vi "Populate Single Control.vi"(5 "Clust Refnum":refnum<vi>, 6 "VI Refnum":refnum<vi>, 7 "Prefix":string, 8 "error in (no error)":errorcluster, 9 "Values":string[](array[string]), 10 "Keys":string[](array[string]), 11 "Ctl Refnum":refnum<vi>) -> (0 "error out":errorcluster, 1 "Variant":variant, 3 "Ctl Refnum out":refnum<vi>, 4 "VI Refnum out":refnum<vi>)   [LabVIEW 2018]
panel:
  in  "type specifier":refnum<vi>
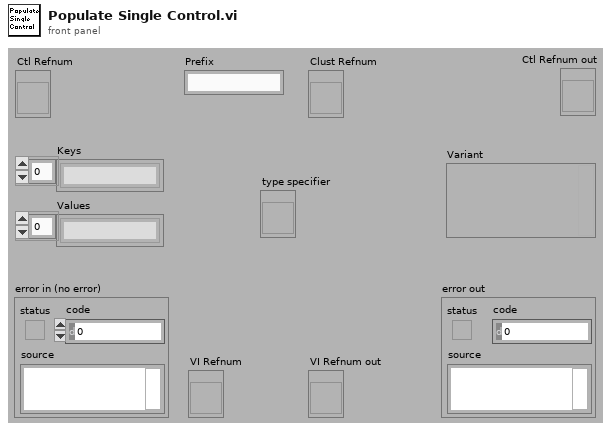
[diagram p1: front panel]
types:
  T1 = typedef "LVComboBoxStrsAndValuesArrayTypeDef.ctl" = cluster{"String":string, "Value":string}[]
  T2 = typedef "LVStringsAndValuesArrayTypeDef.ctl" = cluster{"String":string, "Value":ext}[]
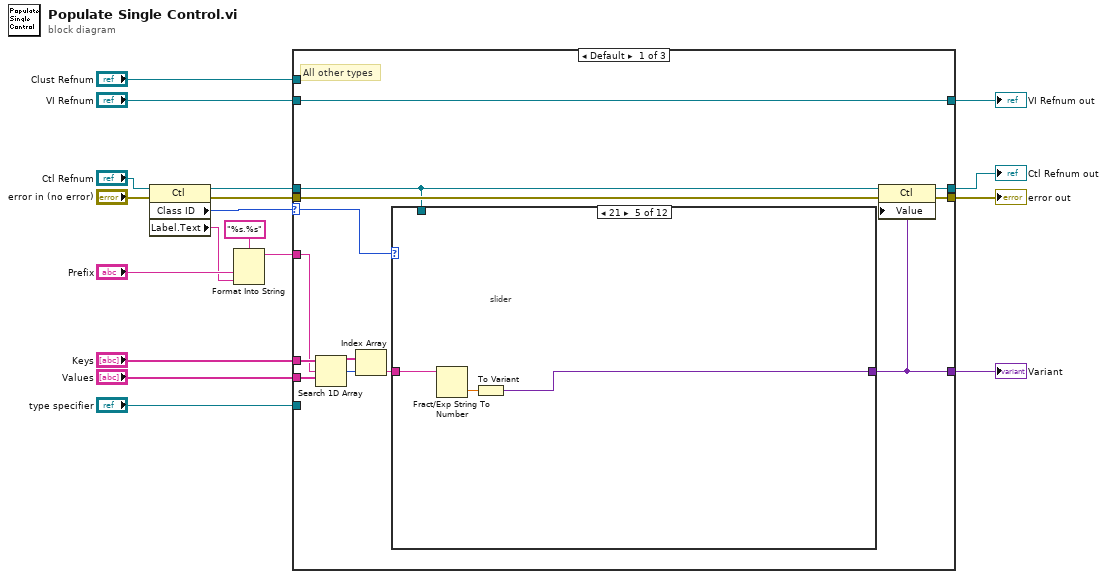
[diagram p0: block diagram]
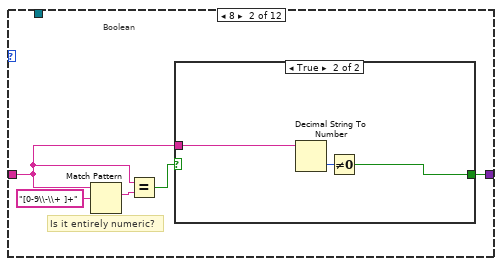
[diagram p3: hidden frame]
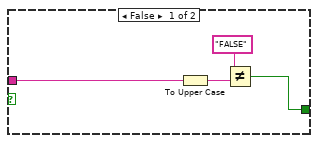
[diagram p4: hidden frame]
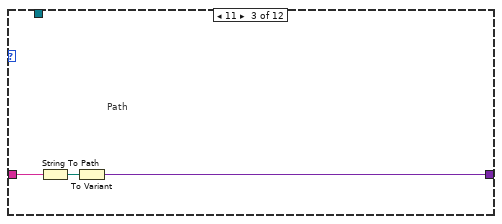
[diagram p5: hidden frame]
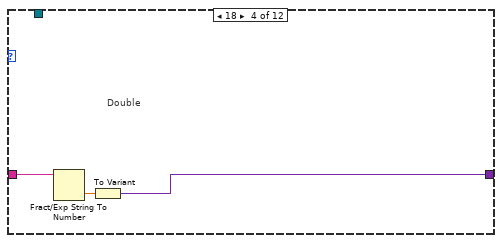
[diagram p6: hidden frame]
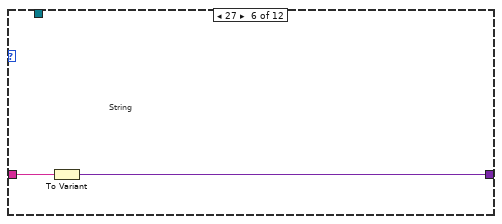
[diagram p7: hidden frame]
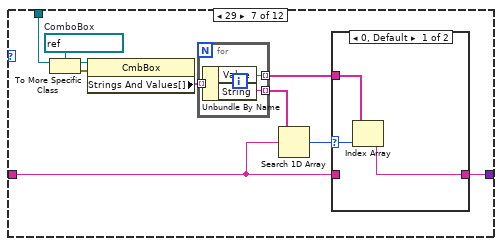
[diagram p8: hidden frame]
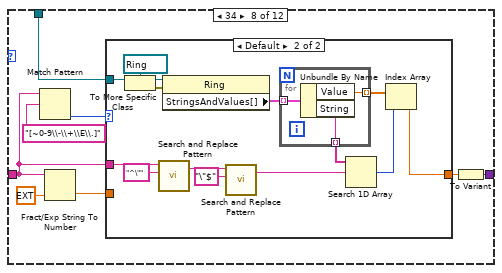
[diagram p10: hidden frame]
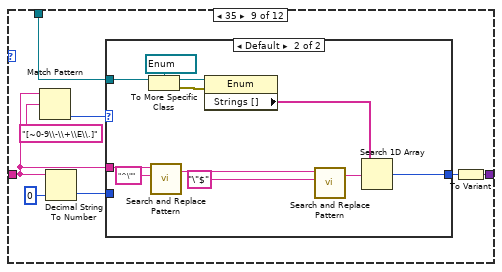
[diagram p12: hidden frame]
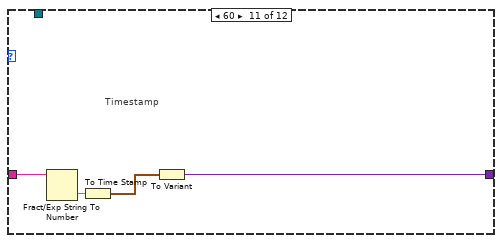
[diagram p15: hidden frame]
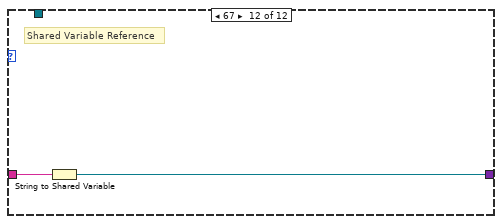
[diagram p16: hidden frame]
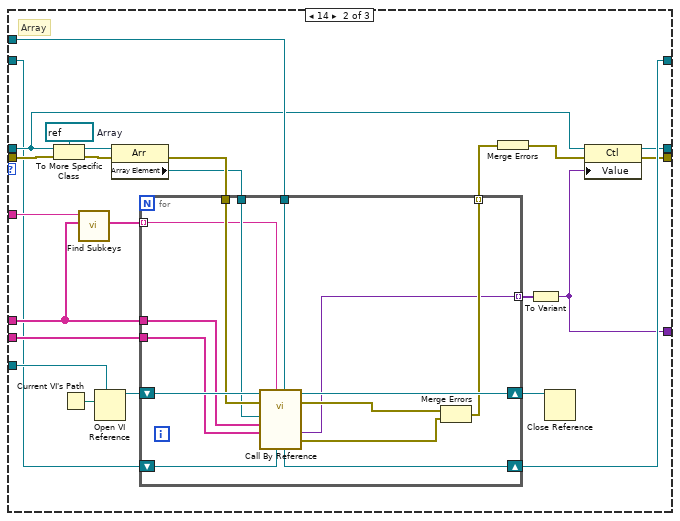
[diagram p17: hidden frame]
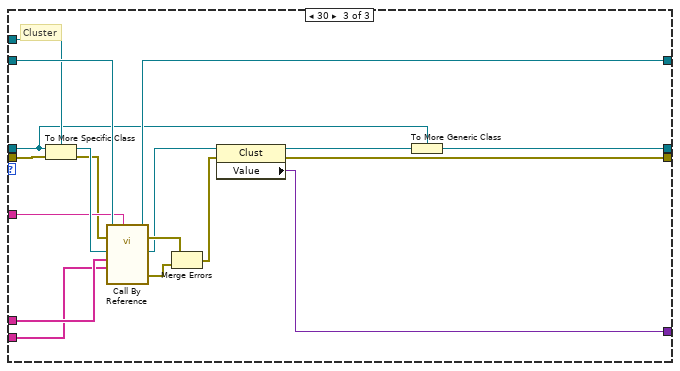
[diagram p18: hidden frame]
diagram:
  n1 = property class="Ctl"(reference="Ctl Refnum", error in="error in (no error)") -> (reference out=w10:refnum<vi>, error out=w11:errorcluster, "Class ID"=w9:u32, "Label.Text"=w6:string)
  n2 = Format Into String(format string="%s.%s", "Prefix", w6) -> (resulting string=w18:string)  [unwired: 2 in, 1 out]
  n3 = case shown="Default" w9 {
    selector: w9 -> [w25 _ _]
    tunnel: "VI Refnum" -> [w26 w125 w178]
    tunnel: w10 -> [w20 w135 w170]
    tunnel: w11 -> [w29 w147 w179]
    tunnel: w18 -> [w19 w132 w173]
    tunnel: "Values" -> [w30 w143 w175]
    tunnel: "Keys" -> [w23 w131 w176]
    tunnel: [w26 w144 w177] -> w14
    tunnel: [w28 w134 w171] -> w17
    tunnel: [w27 w126 w162] -> w16
    tunnel: "Clust Refnum" -> [_ w145 w172]
    tunnel: [w21 w133 w165] -> w3
    tunnel: "type specifier" -> [_ w138 _]
    frame Default {
      # "All other types"
      n4 = Search 1D Array(1D array=w23, element=w19) -> (index of element=w22:i32)  [unwired: 1 in]
      n5 = Index Array(array=w30, index=w22) -> (element=w24:string)
      n6 = case shown="21" w25 {
        tunnel: w24 -> [_ w31 w44 w48 w51 w52 w56 w71 w97 w117 w121 w123]
        tunnel: [_ w32 w45 w46 w49 w53 w55 w77 w103 w117 w120 w122] -> w21
        tunnel: w20 -> [_ _ _ _ _ _ w63 w76 w102 _ _ _]
        frame Default {
        }
        frame 8 {
          # "Is it entirely numeric?"
          # "Boolean"
          n7 = Match Pattern(string=w31, regular expression="[0-9\\-\\+ ]+") -> (match substring=w34:string)  [unwired: 1 in, 3 out]
          n8 = Equal?(x=w31, y=w34) -> (x = y?=w33:bool)
          n9 = case shown="True" w33 {
            tunnel: [w36 w40] -> w32
            tunnel: w31 -> [w37 w42]
            frame False {
              n10 = To Upper Case(1:w37) -> (0:w39:string)
              n11 = Not Equal?(x="FALSE", y=w39) -> (x != y?=w36:bool)
            }
            frame True {
              n12 = Decimal String To Number(string=w42) -> (number=w41:i32)  [unwired: 2 in, 1 out]
              n13 = Not Equal To 0?(x=w41) -> (x != 0?=w40:bool)
            }
          }
        }
        frame 11 {
          # "Path"
          n14 = String To Path(string=w44) -> (path=w43:path)
          n15 = To Variant(anything=w43) -> (Variant=w45:variant)
        }
        frame 18 {
          # "Double"
          n16 = Fract/Exp String To Number(string=w48) -> (number=w47:dbl)  [unwired: 3 in, 1 out]
          n17 = To Variant(anything=w47) -> (Variant=w46:variant)
        }
        frame 21 {
          # "slider"
          n18 = Fract/Exp String To Number(string=w51) -> (number=w50:dbl)  [unwired: 3 in, 1 out]
          n19 = To Variant(anything=w50) -> (Variant=w49:variant)
        }
        frame 27 {
          # "String"
          n20 = To Variant(anything=w52) -> (Variant=w53:variant)
        }
        frame 29 {
          w62 = refnum<vi> refnum  # ComboBox
          n21 = To More Specific Class(target class=w62, reference=w63) -> (specific class reference=w61:refnum<vi>, error out=w60:errorcluster)  [unwired: 1 in]
          n22 = property class="CmbBox"(reference=w61, error in=w60) -> ("Strings And Values[]"=w59:T1)  [unwired: 2 out]
          n23 = for {
            tunnel: w59 -> [w70] mode=indexing
            tunnel: [w69] -> w58 mode=indexing
            tunnel: [w68] -> w54 mode=indexing
            n24 = Unbundle By Name(w70) -> ("Value"=w68:string, "String"=w69:string)
          }
          n25 = Search 1D Array(1D array=w58, element=w56) -> (index of element=w57:i32)  [unwired: 1 in]
          n26 = case shown="0, Default" w57 {
            selector: w57 -> [w65 _]
            tunnel: [w64 w67] -> w55
            tunnel: w56 -> [_ w67]
            tunnel: w54 -> [w66 _]
            frame 0, Default {
              n27 = Index Array(array=w66, index=w65) -> (element=w64:string)
            }
            frame -1 {
            }
          }
        }
        frame 34 {
          n28 = Match Pattern(string=w71, regular expression="[~0-9\\-\\+\\E\\.]") -> (offset past match=w75:i32)  [unwired: 1 in, 3 out]
          n29 = Fract/Exp String To Number(string=w71, default (0 dbl)=ext 0.0 ("default (0 I32)")) -> (number=w73:ext)  [unwired: 2 in, 1 out]
          n30 = case shown="Default" w75 {
            tunnel: w76 -> [_ w90]
            tunnel: [w79 w80] -> w72
            tunnel: w73 -> [w79 _]
            tunnel: w71 -> [_ w88]
            frame -1 {
            }
            frame Default {
              n31 = To More Specific Class(target class=refnum<vi> refnum ("Enum Class"), reference=w90) -> (specific class reference=w93:refnum<vi>, error out=w92:errorcluster)  [unwired: 1 in]
              n32 = call <vilib>:"Search and Replace Pattern.vi"("string"=w88, "regular expression (\"\")"="^\"" ("regular expression (\"\")")) -> ("result string"=w86:string)  [unwired: 3 in, 1 out]
              n33 = property class="Ring"(reference=w93, error in=w92) -> ("StringsAndValues[]"=w84:T2)  [unwired: 2 out]
              n34 = call <vilib>:"Search and Replace Pattern.vi"("string"=w86, "regular expression (\"\")"="\"$" ("regular expression (\"\")")) -> ("result string"=w85:string)  [unwired: 3 in, 1 out]
              n35 = for {
                tunnel: w84 -> [w96] mode=indexing
                tunnel: [w95] -> w82 mode=indexing
                tunnel: [w94] -> w83 mode=indexing
                n36 = Unbundle By Name(w96) -> ("Value"=w95:ext, "String"=w94:string)
              }
              n37 = Search 1D Array(1D array=w83, element=w85) -> (index of element=w81:i32)  [unwired: 1 in]
              n38 = Index Array(array=w82, index=w81) -> (element=w80:ext)
            }
          }
          n39 = To Variant(anything=w72) -> (Variant=w77:variant)
        }
        frame 35 {
          n40 = Match Pattern(string=w97, regular expression="[~0-9\\-\\+\\E\\.]") -> (offset past match=w101:i32)  [unwired: 1 in, 3 out]
          n41 = Decimal String To Number(string=w97, default (0L)=u32 0 ("default (0 I32)")) -> (number=w99:u32)  [unwired: 1 in, 1 out]
          n42 = case shown="Default" w101 {
            tunnel: w102 -> [_ w113]
            tunnel: [w105 w109] -> w98
            tunnel: w99 -> [w105 _]
            tunnel: w97 -> [_ w110]
            frame -1 {
            }
            frame Default {
              n43 = To More Specific Class(target class=refnum<vi> refnum ("Enum Class"), reference=w113) -> (specific class reference=w116:refnum<vi>, error out=w115:errorcluster)  [unwired: 1 in]
              n44 = call <vilib>:"Search and Replace Pattern.vi"("string"=w110, "regular expression (\"\")"="^\"" ("regular expression (\"\")")) -> ("result string"=w107:string)  [unwired: 3 in, 1 out]
              n45 = property class="Enum"(reference=w116, error in=w115) -> ("Strings []"=w112:string[])  [unwired: 2 out]
              n46 = call <vilib>:"Search and Replace Pattern.vi"("string"=w107, "regular expression (\"\")"="\"$" ("regular expression (\"\")")) -> ("result string"=w106:string)  [unwired: 3 in, 1 out]
              n47 = Search 1D Array(1D array=w112, element=w106) -> (index of element=w109:i32)  [unwired: 1 in]
            }
          }
          n48 = To Variant(anything=w98) -> (Variant=w103:variant)
        }
        frame 50 {
        }
        frame 60 {
          # "Timestamp"
          n49 = Fract/Exp String To Number(string=w121) -> (number=w119:dbl)  [unwired: 3 in, 1 out]
          n50 = To Time Stamp(1:w119) -> (0:w118:timestamp)
          n51 = To Variant(anything=w118) -> (Variant=w120:variant)
        }
        frame 67 {
          # "Shared Variable Reference"
          n52 = String to Shared Variable(0:w123) -> (2:w122:refnum<k21>)  [unwired: 1 out]
        }
      }
      n53 = property class="Ctl"(reference=w20, error in=w29, "Value"=w21) -> (reference out=w28:refnum<vi>, error out=w27:errorcluster)
    }
    frame 14 {
      w146 = refnum<vi> refnum  # Array
      # "Array"
      n54 = To More Specific Class(target class=w146, reference=w135, error in=w147) -> (specific class reference=w141:refnum<vi>, error out=w128:errorcluster)
      n55 = Current VI's Path() -> (path=w140:path)
      n56 = call "Find Subkeys.vi"("Keys"=w131, "Key Root"=w132) -> ("Subkeys"=w142:string[])  [unwired: 9 in]
      n57 = Open VI Reference(type specifier VI Refnum (for type only)=w138, vi path=w140) -> (vi reference=w139:refnum<vi>)  [unwired: 4 in, 1 out]
      n58 = property class="Arr"(reference=w141, error in=w128) -> (error out=w130:errorcluster, "Array Element"=w129:refnum<vi>)  [unwired: 1 out]
      n59 = for {
        tunnel: w131 -> [w160]
        tunnel: w143 -> [w159]
        tunnel: w145 -> [w158]
        tunnel: w129 -> [w154]
        tunnel: w130 -> [w155]
        tunnel: [w152] -> w136 mode=indexing
        tunnel: w142 -> [w151] mode=indexing
        shift-right: [w150] -> w144
        shift-left: w125 -> [w149]
        shift-right: [w157] -> w137
        shift-left: w139 -> [w161]
        tunnel: [w148] -> w124 mode=indexing
        n60 = call-by-ref "?"(reference=w161, error in=w155, "Clust Refnum"=w158, "VI Refnum"=w149, "Label.Text"=w151, "Values"=w159, "Keys"=w160, "Ctl Refnum"=w154) -> (reference out=w157:refnum<vi>, error out=w153:errorcluster, 0:"error out"=w156:errorcluster, "Variant"=w148:variant, "VI Refnum out"=w150:refnum<vi>)  [unwired: 2 in, 1 out]
        n61 = Merge Errors(w153, w156) -> (w152:errorcluster)
      }
      n62 = Merge Errors(w136) -> (w127:errorcluster)
      n63 = To Variant(anything=w124) -> (Variant=w133:variant)
      n64 = Close Reference(reference=w137) -> ()  [unwired: 1 in, 1 out]
      n65 = property class="Ctl"(reference=w135, error in=w127, "Value"=w133) -> (reference out=w134:refnum<vi>, error out=w126:errorcluster)
    }
    frame 30 {
      # "Cluster"
      n66 = To More Specific Class(target class=w172, reference=w170, error in=w179) -> (specific class reference=w174:refnum<vi>, error out=w163:errorcluster)
      n67 = call-by-ref "?"(reference=w178, error in=w163, "Prefix Name"=w173, "Values"=w175, "Keys"=w176, "Clust Refnum"=w174) -> (reference out=w177:refnum<vi>, error out=w168:errorcluster, 0:"error out"=w169:errorcluster, "Cluster Refnum (Dup)"=w167:refnum<vi>)  [unwired: 6 in]
      n68 = Merge Errors(w168, w169) -> (w164:errorcluster)
      n69 = property class="Clust"(reference=w167, error in=w164) -> (reference out=w166:refnum<vi>, error out=w162:errorcluster, "Value"=w165:variant)
      n70 = To More Generic Class(target class=w170, reference=w166) -> (generic class reference=w171:refnum<vi>)
    }
  }
  "Ctl Refnum out" <- w17
  "error out" <- w16
  "VI Refnum out" <- w14
  "Variant" <- w3
